vi "Write Cycle period.vi"(8 "error in (no error)":errorcluster, 10 "Cycle period":dbl, 11 "Instrument Driver in":refnum<class "Instrument Driver.lvclass">) -> (0 "error out":errorcluster, 3 "Instrument Driver out":refnum<class "Instrument Driver.lvclass">)   [LabVIEW 2019, in "Instrument Driver.lvclass"]
uses:
  Instrument Driver.lvclass
  Instrument Driver.lvclass/Instrument Driver.ctl
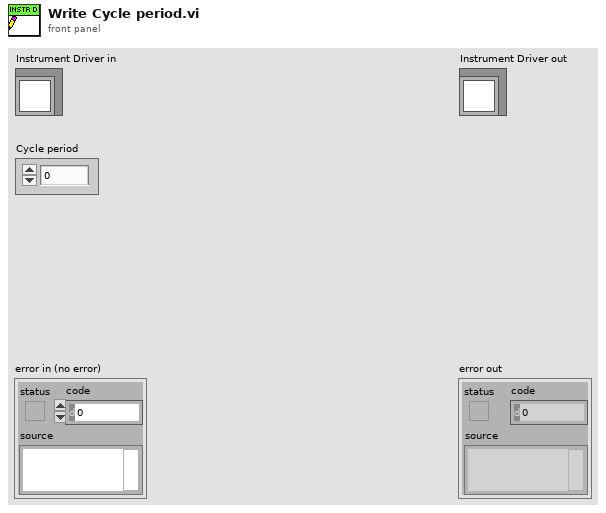
[diagram p1: front panel]
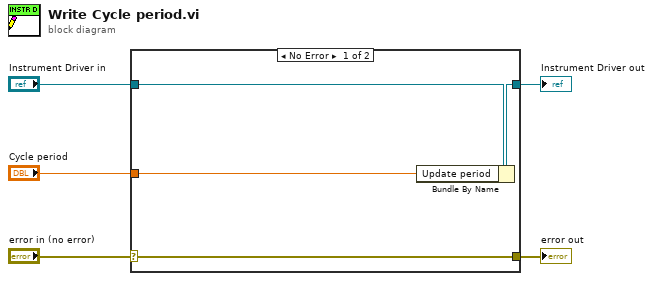
[diagram p0: block diagram]
diagram:
  n1 = case shown="No Error" "error in (no error)" {
    selector: "error in (no error)" -> [w9 w10]
    tunnel: [w9 w10] -> w4
    tunnel: [w7 w11] -> w2
    tunnel: "Instrument Driver in" -> [w8 w11]
    tunnel: "Cycle period" -> [w6 _]
    frame No Error {
      n2 = Bundle By Name(cluster=w8, "Update period"=w6) -> (w7:refnum<class "Instrument Driver.lvclass">)
    }
    frame Error {
    }
  }
  "error out" <- w4
  "Instrument Driver out" <- w2
